vi "PrepareFrames.vi"(9 "Frames Limit":i32, 10 "Frames":i32) -> (2 "FrameList":i32[](array[numeric]))   [LabVIEW 2020]
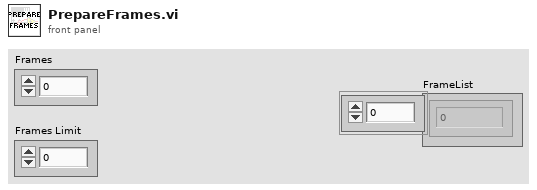
[diagram p1: front panel]
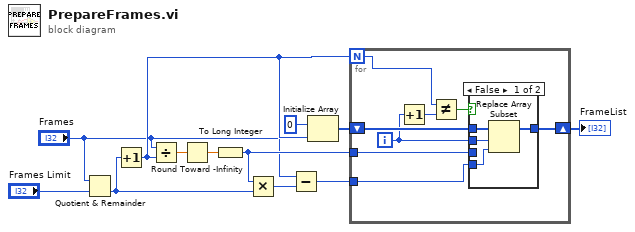
[diagram p0: block diagram]
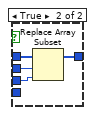
[diagram p2: hidden frame]
diagram:
  n1 = Quotient & Remainder(x="Frames", y="Frames Limit") -> (floor(x/y)=w7:i32)  [unwired: 1 out]
  n2 = Increment(x=w7) -> (x+1=w8:i32)
  n3 = Divide(x="Frames", y=w8) -> (x/y=w12:dbl)
  n4 = Round Toward -Infinity(1:w12) -> (0:w9:dbl)
  n5 = To Long Integer(number=w9) -> (32bit integer=w5:i32)
  n6 = Multiply(x=w5, y=w7) -> (x*y=w6:i32)
  n7 = Subtract(x="Frames", y=w6) -> (x-y=w4:i32)
  n8 = Initialize Array(0, w8) -> (w10:i32[])
  n9 = for {
    N: w8 -> [w19]
    shift-right: [w14] -> w1
    shift-left: w10 -> [w17]
    tunnel: w5 -> [w15]
    tunnel: w4 -> [w13]
    i -> [w16]
    n10 = Increment(x=w16) -> (x+1=w20:i32)
    n11 = Not Equal?(x=w19, y=w20) -> (x != y?=w18:bool)
    n12 = case shown="False" w18 {
      tunnel: w17 -> [w24 w28]
      tunnel: w16 -> [w23 w27]
      tunnel: w15 -> [_ w26]
      tunnel: [w21 w25] -> w14
      tunnel: w13 -> [w22 _]
      frame False {
        n13 = Replace Array Subset(array=w24, new element=w22, index=w23) -> (w21:i32[])
      }
      frame True {
        n14 = Replace Array Subset(array=w28, new element=w26, index=w27) -> (w25:i32[])
      }
    }
  }
  "FrameList" <- w1
